vi "oa_Create Indice Save Last Element.vi"(1 "time":dbl[](array[numeric]), 4 "speed":dbl[](array[numeric]), 6 "reset":bool) -> (14 "first time element":dbl, 15 "last time element":dbl, 16 "time output":dbl[](array[numeric]), 17 "first speed element":dbl, 18 "last speed element":dbl, 19 "speed output":dbl[](array[numeric]))   [LabVIEW 2017, in "SoundVib_OAUtility.lvlib"]
uses:
  <vilib>/addons/Sound and Vibration/Order Analysis/Utility/SoundVib_OAUtility.lvlib
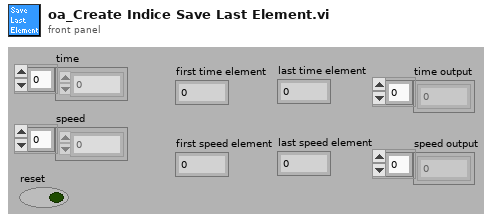
[diagram p1: front panel]
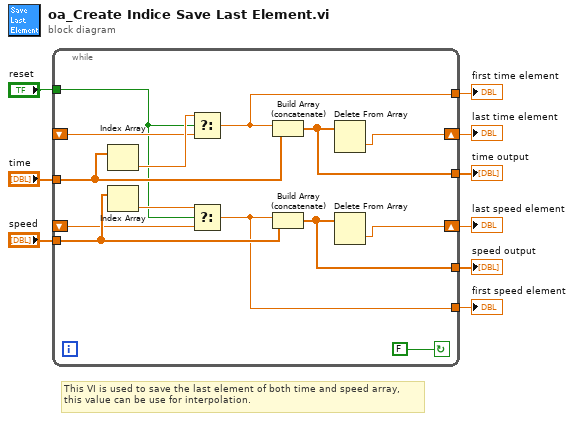
[diagram p0: block diagram]
diagram:
  # "This VI is used to save the last element of both time and speed array,\nthis value can be use for interpolation."
  n1 = while {
    tunnel: "time" -> [w21]
    tunnel: "speed" -> [w20]
    shift-right: [w14] -> w4
    shift-left: _ -> [w18]
    shift-right: [w15] -> w3
    shift-left: _ -> [w17]
    tunnel: "reset" -> [w16]
    tunnel: [w13] -> w6
    tunnel: [w12] -> w5
    tunnel: [w11] -> w2
    tunnel: [w10] -> w1
    stop <- FALSE continue-if-true
    n2 = Index Array(array=w21) -> (element=w23:dbl)  [unwired: 1 in]
    n3 = Index Array(array=w20) -> (element=w22:dbl)  [unwired: 1 in]
    n4 = Select(t=w23, s=w16, f=w18) -> (s? t:f=w11:dbl)
    n5 = Select(t=w22, s=w16, f=w17) -> (s? t:f=w10:dbl)
    n6 = Build Array (concatenate)(w11, w21) -> (w13:dbl[])
    n7 = Build Array (concatenate)(w10, w20) -> (w12:dbl[])
    n8 = Delete From Array(array=w13) -> (deleted portion=w14:dbl)  [unwired: 2 in, 1 out]
    n9 = Delete From Array(array=w12) -> (deleted portion=w15:dbl)  [unwired: 2 in, 1 out]
  }
  "time output" <- w6
  "speed output" <- w5
  "last time element" <- w4
  "last speed element" <- w3
  "first time element" <- w2
  "first speed element" <- w1
